vi "Sr830sens_giulia.vi"(1 "Sr 830 sensitivity":T1(ring), 2 "Change sensitivity ?":bool, 3 "SR830":refnum<visa-resource-name>="GPIB0::24::INSTR") -> (0 "Current Sr 830 sensitivity":T1(ring))   [LabVIEW 2011]
panel:
  out "chaîne concaténée":string
  out "Sensitivity":string
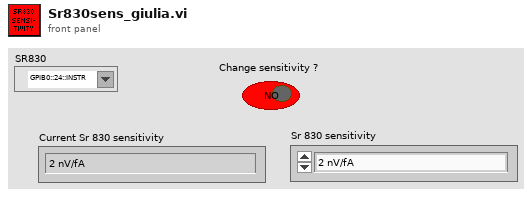
[diagram p1: front panel]
types:
  T1 = enum16{"2 nV/fA", "5 nV/fA", "10 nV/fA", "20 nV/fA", "50 nV/fA", "100 nV/fA", "200 nV/fA", "500 nV/fA", "1 uV/pA", "2 uV/pA", "5 uV/pA", "10 uV/pA", "20 uV/pA", "50 uV/pA", "100 uV/pA", "200 uV/pA", "500 uV/pA", "1 mV/nA", "2 mV/nA", "5 mV/nA", "10 mV/nA", "20 mV/nA", "50 mV/nA", "100 mV/nA", "200 mV/nA", "500 mV/nA", "1 V/uA"}
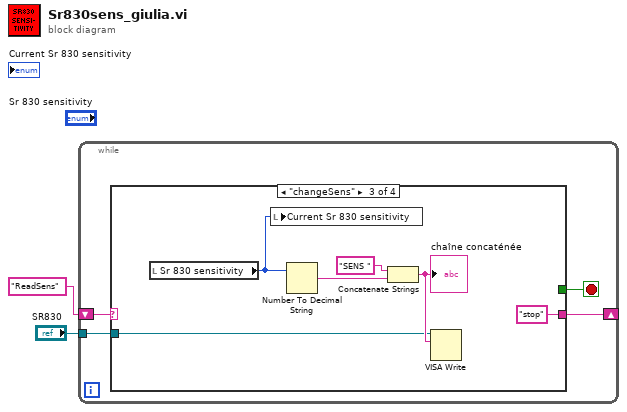
[diagram p0: block diagram]
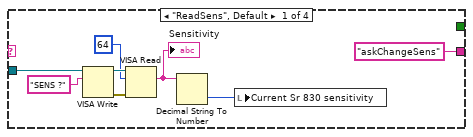
[diagram p2: hidden frame]
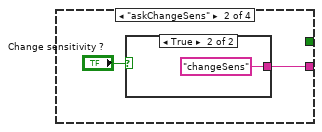
[diagram p3: hidden frame]
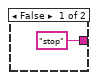
[diagram p4: hidden frame]
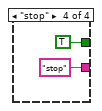
[diagram p5: hidden frame]
diagram:
  n1 = while {
    tunnel: "SR830" -> [w6]
    shift-right: [w5] -> _
    shift-left: "ReadSens" -> [w4]
    stop <- w3 stop-if-true
    n2 = case shown="\"changeSens\"" w4 {
      tunnel: w6 -> [w10 _ w20 _]
      tunnel: ["askChangeSens" w16 "stop" "stop"] -> w5
      tunnel: [_ _ _ TRUE] -> w3
      frame "ReadSens", Default {
        n3 = VISA Write(VISA resource name=w10, write buffer="SENS ?" ("Command")) -> (VISA resource name out=w13:refnum<visa-resource-name>, error out=w12:errorcluster)  [unwired: 1 in, 1 out]
        n4 = VISA Read(VISA resource name=w13, byte count=u32 64 ("nombre d'octets"), error in (no error)=w12) -> (read buffer=w9:string)  [unwired: 3 out]
        "Sensitivity" <- w9
        n5 = Decimal String To Number(string=w9) -> (number=w7:i32)  [unwired: 2 in, 1 out]
        n6 = local write "Current Sr 830 sensitivity"(w7) -> ()
      }
      frame "askChangeSens" {
        n7 = case shown="True" "Change sensitivity ?" {
          tunnel: ["stop" "changeSens"] -> w16
          frame False {
          }
          frame True {
          }
        }
      }
      frame "changeSens" {
        n8 = local read "Sr 830 sensitivity"() -> (w19:T1)
        n9 = local write "Current Sr 830 sensitivity"(w19) -> ()
        n10 = Number To Decimal String(number=w19) -> (decimal integer string=w23:string)  [unwired: 1 in]
        n11 = Concatenate Strings("SENS " ("chaîne"), w23) -> (w21:string)
        "chaîne concaténée" <- w21
        n12 = VISA Write(VISA resource name=w20, write buffer=w21) -> ()  [unwired: 1 in, 3 out]
      }
      frame "stop" {
      }
    }
  }
